vi "Main Editor UI.vi"() -> ()   [LabVIEW 2015, in "SystemLink File editor node.lvclass"]
doc: "This is the main view for configuration the behavior of a module in the DCAF standard editor."
uses:
  SystemLink File editor node.lvclass
  <vilib>/NI/Configuration Framework/Controls/EventCluster.ctl
  <vilib>/NI/Configuration Framework/NISE_CEF_TreeControl.lvlib
  <vilib>/NI/Configuration Framework/Node/UserEventRef.ctl
  <vilib>/NI/Configuration Framework/Node/NISE_CEF_Node.lvclass
  <vilib>/NI/Tools/Keyed Array/KeyedArray.ctl
  <vilib>/NI/Tools/Keyed Array/Tools_KeyedArray.lvlib
  <vilib>/NI/AMC/Message.ctl
  <vilib>/NI/AMC/AMC.lvlib
  <vilib>/NI/AMC/Message Queue.ctl
  <vilib>/NI/Tag Bus/tag/tag descriptor.lvclass
  <vilib>/NI/Tag Bus Module Framework/channel/TBM channel.lvclass
  <vilib>/NI/DCAF/Tag Editor Core/Table API/Available Tag Menu/channel action event.ctl
  <vilib>/NI/DCAF/Tag Editor Core/Table API/Table Manager.lvlib
  <vilib>/NI/Configuration Framework/Node/NodeRef.ctl
  <vilib>/NI/Configuration Framework/Node/NodeChangeEvent.ctl
  <vilib>/NI/Configuration Framework/Node/CacheState.ctl
  <vilib>/NI/Configuration Framework/Node/RefreshUIEvent.ctl
  <vilib>/NI/Configuration Framework/Node/StopEvent.ctl
  <vilib>/NI/DCAF/Tag Editor Core/Table API/Table Manager/references.ctl
  <vilib>/NI/DCAF/Tag Editor Core/Table API/Table Manager/Table Manager.lvclass
  <vilib>/NI/DCAF/Tag Editor Core/Table API/Listbox/Multi Column Listbox.lvclass
  <vilib>/Utility/miscctls.llb/LVPositionTypeDef.ctl
  <vilib>/NI/DCAF UI Toolkit/Controls/DCAF UI Elements.lvlib
  <vilib>/NI/DCAF/Tag Editor Core/Table API/Table Manager/Call Back Ref Type Def.ctl
  <vilib>/NI/DCAF/Tag Editor Core/Table API/Available Tag Menu/dialog output action.ctl
  module/configuration/SystemLink File configuration.lvclass
  <vilib>/NI/DCAF/Tag Editor Core/Configuration Editor/Classes/Engine Parent/Engine Parent Editor Node.lvclass
  <vilib>/NI/DCAF/Tag Editor Core/Configuration Editor/Classes/Module editor node/module editor node.lvclass
  module/configuration/Permissions Enum.ctl
  <vilib>/NI/DCAF UI Toolkit/Controls/Import.ctl
  <vilib>/NI/DCAF UI Toolkit/Controls/Export.ctl
  module/configuration/Data Tag Type.ctl
panel:
  in  "Data Type":T1
  in  "user event out":refnum<user-event>
  in  "Permissions":T2
  in  "node change":T3
  in  "cache state":T4
  in  "refresh UI":T5
  in  "stop event":T6
  in  "Tab Control":T7(tab)=enum."Connection Configuration"
  in  "Table":i32(listbox)
  in  "Configuration":T8={"Configuration ID"="", "HTTP"={"Verify Server?"=TRUE, "Server URL"="", "CA Certificate File"="", "User Info"={"Username"="", "Password"=""}, "API Key"=""}}
  in  "Connection Type":T9(ring)
  in  "Export":T10
  in  "Import":T11
  in  "user event":T12
  in  "main queue":T13
  in  "node ref":T14
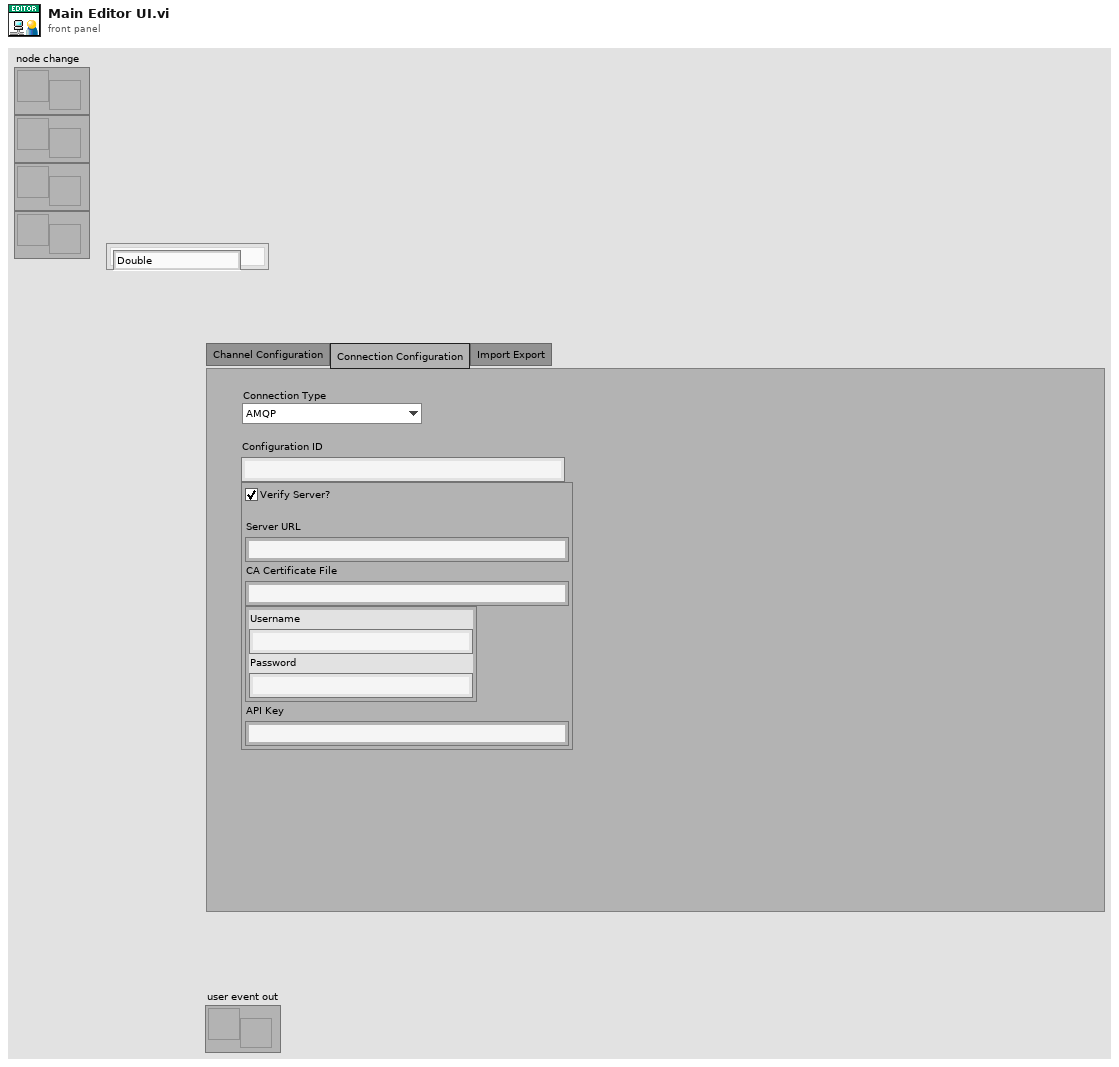
[diagram p1: front panel]
types:
  T1 = typedef "SystemLink File configuration.lvclass/Data Tag Type.ctl" = enum16{"Double", "Single", "I32", "I16", "I8", "U64", "U32", "U16", "U8", "Boolean", "String", "Timestamp"}
  T2 = typedef "SystemLink File configuration.lvclass/Permissions Enum.ctl" = enum16{"Read from SystemLink", "Write to SystemLink"}
  T3 = typedef "NISE_CEF_Node.lvclass/NodeChangeEvent.ctl" = refnum<user-event>
  T4 = typedef "NISE_CEF_Node.lvclass/CacheState.ctl" = refnum<user-event>
  T5 = typedef "NISE_CEF_Node.lvclass/RefreshUIEvent.ctl" = refnum<user-event>
  T6 = typedef "NISE_CEF_Node.lvclass/StopEvent.ctl" = refnum<user-event>
  T7 = enum32{"Channel Configuration", "Connection Configuration", "Import Export"}
  T8 = cluster{"Configuration ID":string, "HTTP":cluster{"Verify Server?":bool, "Server URL":string, "CA Certificate File":string, "User Info":cluster{"Username":string, "Password":string}, "API Key":string}}
  T9 = enum16{"AMQP", "HTTP", "API Key (SystemLink Cloud)"}
  T10 = typedef "DCAF UI Elements.lvlib/Export.ctl" = bool
  T11 = typedef "DCAF UI Elements.lvlib/Import.ctl" = bool
  T12 = typedef "NISE_CEF_Node.lvclass/UserEventRef.ctl" = refnum<user-event>
  T13 = typedef "AMC.lvlib/Message Queue.ctl" = refnum<queue>
  T14 = typedef "NISE_CEF_Node.lvclass/NodeRef.ctl" = refnum<data-value>
  T15 = typedef "Table Manager.lvlib/Table Manager.lvclass/references.ctl" = cluster{"stop event":T6, "refresh UI":T5, "cache state":T4, "node change":T3, "user event out":refnum<user-event>, "main queue":T13, "user event":T12}
  T16 = typedef "LVPositionTypeDef.ctl" = cluster{"Left":i32, "Top":i32}
  T17 = typedef "Table Manager.lvlib/Table Manager.lvclass/object ref.ctl" = cluster{"engine":refnum<data-value>, "Node Ref":refnum<data-value>}
  T18 = typedef "Table Manager.lvlib/Column.lvclass/Column Descriptor.ctl" = cluster{"name":string, "caption":string, "Column Type":T19, "Params":string, "AutoSizeMode":i32, "FillWeight":sgl, "MinWidth":u32, "tooltip":string, "Enum Reference":refnum<vi>, "Channel suffix":string, "Read Only":bool, "Call Back VI":T20, "DT Dependency":i32, "name dependency":i32, "data type":T21, "Custom Column":refnum<class "Column.lvclass">}
  T19 = typedef "Table Manager.lvlib/Column.lvclass/Column Type.ctl" = enum16{"String", "Mapping", "Enum", "Custom"}
  T20 = typedef "Table Manager.lvlib/Table Manager.lvclass/Call Back Ref Type Def.ctl" = refnum<vi>
  T21 = typedef "tag bus.lvlib/tag descriptor.lvclass/Data Type.ctl" = enum16{"Double", "Single", "I64", "I32", "I16", "I8", "U64", "U32", "U16", "U8", "Boolean", "String", "Array of Double", "Array of Single", "Array of I64", "Array of I32", "Array of I16", "Array of I8", "Array of U64", "Array of U32", "Array of U16", "Array of U8", "Array of Boolean", "Array of String"}
  T22 = typedef "SystemLink configuration.lvclass/Connection Configuration.ctl" = cluster{"Connection Type":T23, "AMQP":cluster{"Configuration ID":string}, "HTTP":cluster{"Verify Server?":bool, "Server URL":string, "CA Certificate File":string, "User Info":cluster{"Username":string, "Password":string}, "API Key":string}}
  T23 = typedef "SystemLink configuration.lvclass/Connection Type.ctl" = enum16{"AMQP", "HTTP", "API Key (SystemLink Cloud)"}
  T24 = cluster{"Verify Server?":bool, "Server URL":string, "CA Certificate File":string, "User Info":cluster{"Username":string, "Password":string}, "API Key":string}
  T25 = typedef "Table Manager.lvlib/Table Manager.lvclass/Table Events.ctl" = cluster{"Menu Selection":refnum<user-event>}
  T26 = enum8{"Enabled", "Disabled", "Disabled and Grayed Out"}
  T27 = cluster{"AMQP Specific":refnum<vi>, "HTTP Generic":refnum<vi>, "HTTP Specific":refnum<vi>, "API Key Specific":refnum<vi>}
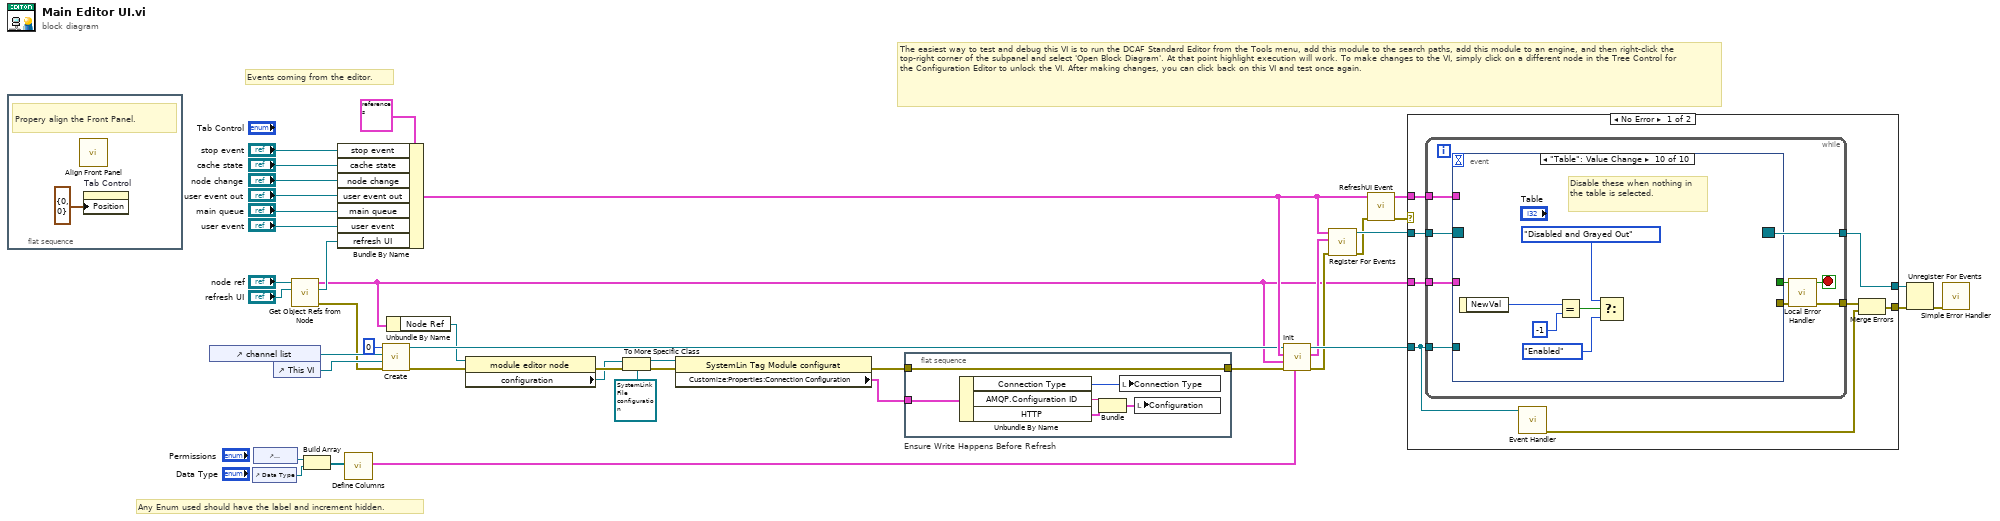
[diagram p0: block diagram]
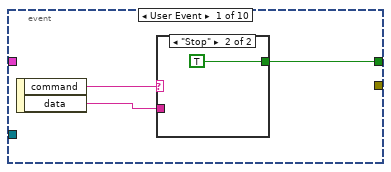
[diagram p2: hidden frame]
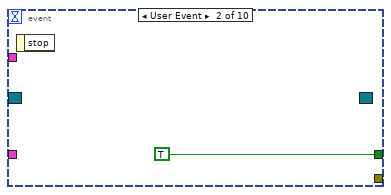
[diagram p4: hidden frame]
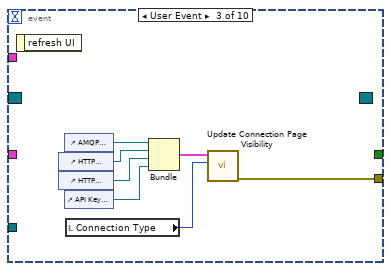
[diagram p5: hidden frame]
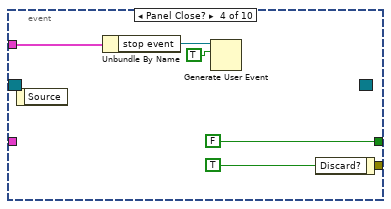
[diagram p6: hidden frame]
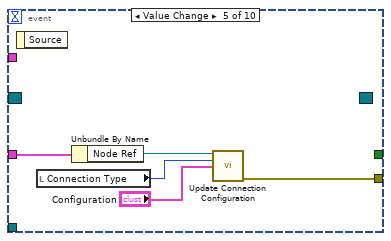
[diagram p7: hidden frame]
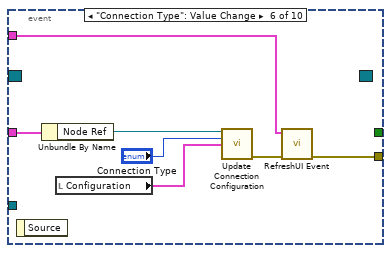
[diagram p8: hidden frame]
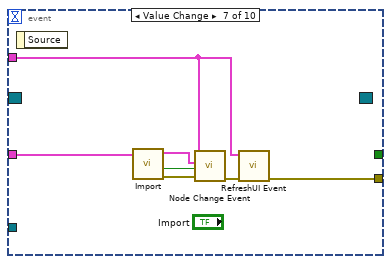
[diagram p9: hidden frame]
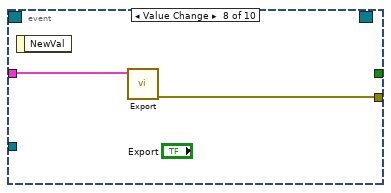
[diagram p10: hidden frame]
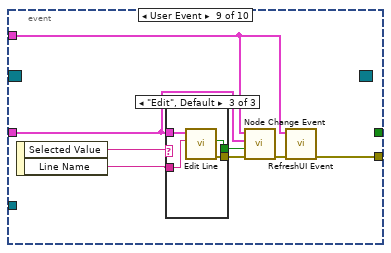
[diagram p11: hidden frame]
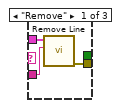
[diagram p12: hidden frame]
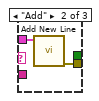
[diagram p13: hidden frame]
diagram:
  # "The easiest way to test and debug this VI is to run the DCAF Standard Editor from the Tools menu, add this module to the search paths, add this module to an engine, and then right-click the top-right corner of the subpanel and select 'Open Block Diagram'. At that point highlight execution will work. To make changes to the VI, simply click on a different node in the Tree Control for the Configuration Editor to unlock the VI. After making changes, you can click back on this VI and test once again."
  # "Any Enum used should have the label and increment hidden."
  # "Events coming from the editor."
  n1 = flat-sequence {
    frame #0 {
      # "Propery align the Front Panel."
      n2 = call <vilib>:"Align Front Panel.vi"() -> ()  [unwired: 10 in, 2 out]
      n3 = property on="Tab Control" class="TabCtl (strict)"("Position"=T16 {"Left"=0, "Top"=0}) -> ()  [unwired: 2 in, 2 out]
    }
  }
  n4 = control-ref of="channel list"() -> (w19:refnum<vi>)
  n5 = control-ref of="Data Type"() -> (w11:refnum<vi>)
  n6 = control-ref of="Permissions"() -> (w27:refnum<vi>)
  n7 = control-ref of="This VI"() -> (w17:refnum<vi>)
  n8 = call "Get Object Refs from Node.vi"("Refresh UI"="refresh UI", "Data Value Reference in"="node ref") -> ("error out"=w14:errorcluster, "Refresh UI out"=w12:T5, "References"=w9:T17)  [unwired: 7 in]
  n9 = Build Array(w27, w11) -> (w26:refnum<vi>[])
  n10 = Bundle By Name(cluster=T15 {"stop event"=refnum, "refresh UI"=refnum, "cache state"=refnum, "node change"=refnum, "user event out"=refnum, "main queue"=refnum, "user event"=refnum} ("References"), "stop event"="stop event", "cache state"="cache state", "node change"="node change", "user event out"="user event out", "main queue"="main queue", "user event"="user event", "refresh UI"=w12) -> (w28:T15)
  n11 = call "Define Columns.vi"("Enum Array"=w26) -> ("Column Definition"=w30:T18[])  [unwired: 10 in]
  n12 = call <vilib>:"Create.vi"("error in (no error)"=w14, "Top VI"=w17, "Listbox"=w19, "Index"=0) -> ("error out"=w15:errorcluster, "reference out"=w16:refnum<class "Multi Column Listbox.lvclass">)  [unwired: 6 in]
  n13 = Unbundle By Name(w9) -> ("Node Ref"=w8:refnum<data-value>)
  n14 = property class="module editor node"(reference=w8, error in=w15) -> (error out=w10:errorcluster, "configuration"=w6:refnum<class "NISE_CEF_serializable configuration.lvclass">)  [unwired: 1 out]
  n15 = To More Specific Class(target class=refnum<class "SystemLink File configuration.lvclass"> refnum ("SystemLin Tag Module configuration"), reference=w6, error in=w10) -> (specific class reference=w4:refnum<class "SystemLink File configuration.lvclass">, error out=w7:errorcluster)
  n16 = property class="SystemLin Tag Module configurat"(reference=w4, error in=w7) -> (error out=w2:errorcluster, "Customize:Properties:Connection Configuration"=w3:T22)  [unwired: 1 out]
  n17 = flat-sequence "Ensure Write Happens Before Refresh" {
    tunnel: w3 -> [w48]
    tunnel: w2 -> [w46]
    tunnel: [w46] -> w1
    frame #0 {
      n18 = Unbundle By Name(w48) -> ("Connection Type"=w47:T23, "AMQP.Configuration ID"=w44:string, "HTTP"=w43:T24)
      n19 = Bundle("Configuration ID"=w44, "HTTP"=w43) -> (w45:T8)  [unwired: 1 in]
      n20 = local write "Connection Type"(w47) -> ()
      n21 = local write "Configuration"(w45) -> ()
    }
  }
  n22 = call-dynamic "Init.vi"("Column Descriptors"=w30, "error in (no error)"=w1, "Node object refs"=w9, "Event References"=w28, "Multi Column Listbox in"=w16) -> ("error out"=w21:errorcluster, "Table Events"=w20:T25, "Multi Column Listbox out"=w25:refnum<class "Multi Column Listbox.lvclass">)  [unwired: 4 in]
  n23 = call "Register For Events.vi"("error in"=w21, "Table Events"=w20, "References"=w28) -> ("error out"=w23:errorcluster, "Event Registration Refnum"=w31:refnum<event-registration>)  [unwired: 7 in]
  n24 = call "RefreshUI Event.vi"("error in (no error)"=w23, "References in"=w28) -> ("error out"=w22:errorcluster, "References out"=w29:T15)  [unwired: 8 in]
  n25 = case shown="No Error" w22 {
    selector: w22 -> [_ w127]
    tunnel: w31 -> [w56 w126]
    tunnel: [w55 w126] -> w41
    tunnel: [w49 w127] -> w40
    tunnel: w29 -> [w54 _]
    tunnel: w9 -> [w53 _]
    tunnel: w25 -> [w52 _]
    frame No Error {
      n26 = while {
        tunnel: w56 -> [w65]
        tunnel: [w64] -> w55
        tunnel: [w61] -> w50
        tunnel: w54 -> [w59]
        tunnel: w53 -> [w58]
        tunnel: w52 -> [w57]
        stop <- w63 stop-if-true
        n27 = event shown="[9] \"Table\": Value Change" {
          selector: w65 -> [_ _ _ _ _ _ _ _ _ _]
          dyn-events: [_ _ _ _ _ _ _ _ _ _] -> w64
          timeout: _ -> [_ _ _ _ _ _ _ _ _ _]
          tunnel: [w68 TRUE _ FALSE _ _ _ _ _ _] -> w62
          tunnel: [_ _ w71 _ w85 w90 w100 w103 w109 _] -> w60
          tunnel: w59 -> [_ _ _ w79 _ w89 w97 _ w105 _]
          tunnel: w58 -> [_ _ _ _ w87 w93 w99 w102 w106 _]
          tunnel: w57 -> [_ _ _ _ _ _ _ _ _ _]
          event User Event {
            n28 = event-data() -> ("command"=w67:string, "data"=w66:string)  [unwired: 1 in]
            n29 = case shown="\"Stop\"" w67 {
              tunnel: [_ TRUE] -> w68
              tunnel: w66 -> [_ _]
              frame Default {
              }
              frame "Stop" {
              }
            }
          }
          event User Event {
            n30 = event-data() -> ()  [unwired: 1 in, 1 out]
          }
          event User Event {
            n31 = event-data() -> ()  [unwired: 1 in, 1 out]
            n32 = control-ref of="HTTP Generic"() -> (w76:refnum<vi>)
            n33 = control-ref of="HTTP Specific"() -> (w75:refnum<vi>)
            n34 = control-ref of="AMQP Specific"() -> (w77:refnum<vi>)
            n35 = control-ref of="API Key Specific"() -> (w74:refnum<vi>)
            n36 = local read "Connection Type"() -> (w72:T9)
            n37 = Bundle("AMQP Specific"=w77, "HTTP Generic"=w76, "HTTP Specific"=w75, "API Key Specific"=w74) -> (w73:T27)  [unwired: 1 in]
            n38 = call "Update Connection Page Visibility.vi"("Connection Type"=w72, "Config References"=w73) -> ("error out"=w71:errorcluster)  [unwired: 9 in]
          }
          event Panel Close? {
            n39 = event-data() -> ()  [unwired: 1 in, 1 out]
            n40 = Unbundle By Name(w79) -> ("stop event"=w78:T6)
            n41 = Generate User Event(user event=w78, event data cluster=TRUE ("event data")) -> ()  [unwired: 2 in, 2 out]
            n42 = event-data("Discard?"=TRUE) -> ()  [unwired: 1 in, 1 out]
          }
          event "Configuration.HTTP", "Configuration.Configuration ID": Value Change {
            n43 = event-data() -> ()  [unwired: 1 in, 1 out]
            n44 = local read "Connection Type"() -> (w84:T9)
            n45 = Unbundle By Name(w87) -> ("Node Ref"=w86:refnum<data-value>)
            n46 = call "Update Connection Configuration.vi"("Data Value Reference in"=w86, "Connection Type"=w84, "Configuration"="Configuration") -> ("error out"=w85:errorcluster)  [unwired: 12 in]
          }
          event "Connection Type": Value Change {
            n47 = event-data() -> ()  [unwired: 1 in, 1 out]
            n48 = Unbundle By Name(w93) -> ("Node Ref"=w94:refnum<data-value>)
            n49 = local read "Configuration"() -> (w88:T8)
            n50 = call "Update Connection Configuration.vi"("Data Value Reference in"=w94, "Connection Type"="Connection Type", "Configuration"=w88) -> ("error out"=w91:errorcluster)  [unwired: 12 in]
            n51 = call "RefreshUI Event.vi"("error in (no error)"=w91, "References in"=w89) -> ("error out"=w90:errorcluster)  [unwired: 8 in, 1 out]
          }
          event Value Change {
            n52 = event-data() -> ()  [unwired: 1 in, 1 out]
            n53 = call "Import.vi"("Objects in"=w99) -> ("error out"=w96:errorcluster, "Update"=w95:bool, "Objects out"=w98:T17)  [unwired: 8 in]
            n54 = call "Node Change Event.vi"("error in (no error)"=w96, "Send (T)"=w95, "objects"=w98, "References in"=w97) -> ("error out"=w101:errorcluster)  [unwired: 7 in]
            n55 = call "RefreshUI Event.vi"("error in (no error)"=w101, "References in"=w97) -> ("error out"=w100:errorcluster)  [unwired: 8 in, 1 out]
          }
          event Value Change {
            n56 = event-data() -> ()  [unwired: 1 in, 1 out]
            n57 = call "Export.vi"("Objects"=w102) -> ("error out"=w103:errorcluster)  [unwired: 10 in]
          }
          event User Event {
            n58 = event-data() -> ("Selected Value"=w111:string, "Line Name"=w108:string)  [unwired: 1 in]
            n59 = case shown="\"Edit\", Default" w111 {
              tunnel: w108 -> [w114 _ w120]
              tunnel: w106 -> [w113 w116 w119]
              tunnel: [w112 w115 w118] -> w107
              tunnel: [_ _ w117] -> w104
              frame "Remove" {
                n60 = call "Remove Line.vi"("Active Line Name"=w114, "Objects"=w113) -> ("error out"=w112:errorcluster)  [unwired: 9 in]
              }
              frame "Add" {
                n61 = call "Add New Line.vi"("objects"=w116) -> ("error out"=w115:errorcluster)  [unwired: 8 in, 2 out]
              }
              frame "Edit", Default {
                n62 = call "Edit Line.vi"("Line Name"=w120, "References"=w119) -> ("error out"=w118:errorcluster, "change?"=w117:bool)  [unwired: 8 in]
              }
            }
            n63 = call "Node Change Event.vi"("error in (no error)"=w107, "Send (T)"=w104, "objects"=w106, "References in"=w105) -> ("error out"=w110:errorcluster)  [unwired: 7 in]
            n64 = call "RefreshUI Event.vi"("error in (no error)"=w110, "References in"=w105) -> ("error out"=w109:errorcluster)  [unwired: 8 in, 1 out]
          }
          event "Table": Value Change {
            # "Disable these when nothing in the table is selected."
            n65 = event-data() -> ("NewVal"=w125:i32)  [unwired: 1 in]
            n66 = Equal?(x=w125, y=-1) -> (x = y?=w123:bool)
            n67 = Select(t=T26."Disabled and Grayed Out" ("Disabled"), s=w123, f=T26."Enabled") -> ()  [unwired: 1 out]
          }
        }
        n68 = call "Local Error Handler.vi"("error in"=w60, "Stop in"=w62) -> ("error out"=w61:errorcluster, "Stop out"=w63:bool)  [unwired: 8 in]
      }
      n69 = call-dynamic "Event Handler.vi"("Listbox in"=w52) -> ("error out"=w51:errorcluster)  [unwired: 9 in, 1 out]
      n70 = Merge Errors(w50, w51) -> (w49:errorcluster)
    }
    frame Error {
    }
  }
  n71 = Unregister For Events(event registration refnum=w41, error in=w40) -> (error out=w39:errorcluster)
  n72 = call <vilib>:"Simple Error Handler.vi"("error in (no error)"=w39) -> ()  [unwired: 4 in, 5 out]
